vi "Auton.vi"(11 "Auton Array":dbl[][](array[numeric])) -> ()   [LabVIEW 2016]
uses:
  Robot Global Data.vi
panel:
  out "Setpoint":dbl
  out "Arg 3":dbl
  out "Arg 1":dbl=0.008
  out "Arg 2":dbl=0.00025
  out "Drive Speed":dbl
  out "Time Left":dbl
  in  "Action Variables":enum32{"Idle - 0", "Driving - 1", "Turning - 2"}(tab)
  in  "Turning Speed Bias":dbl
  in  "Min Turn Speed":dbl
  out "Turn Error":dbl
  in  "Angle Threshold":dbl=1.0
  in  "Max Turn Speed":dbl=0.3
  out "Turn Current":dbl
  out "Step Start Time":u32
  out "Step":i32
  # "Local Variables"
  # "Auton CSV (tab) Format -\n\n(Action)\\t      (Setpoint)\\t       (Timeout)\\t        (Var 1)\\t         (Var 2)\\t         (Var 3)\\t\n\n2       90       10000       0       0       0"
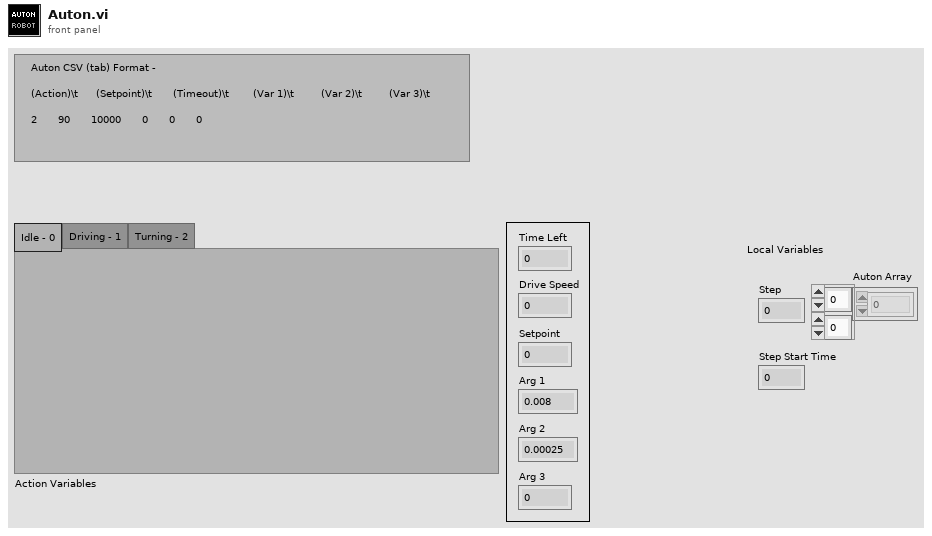
[diagram p1: front panel]
types:
  T1 = typedef "WPI_MotorControlDeviceRef.ctl" = cluster{"DeviceStatus":errorcluster, "Type":T2, "PWM":cluster{"PWM Channel":T3, "DeadBand":T4}, "CAN":cluster{"Device Number":u8, "SetOutput VI Ref":variant, "GetOutput VI Ref":variant, "Enable VI Ref":variant, "Disable VI Ref":variant, "Data":variant}, "Invert":bool}
  T2 = typedef "WPI_MotorControlType.ctl" = enum16{"PWM", "CAN"}
  T3 = typedef "FPGA_DIOPWMChannel.ctl" = enum8{"PWM 0", "PWM 1", "PWM 2", "PWM 3", "PWM 4", "PWM 5", "PWM 6", "PWM 7", "PWM 8", "PWM 9", "PWM MXP 0", "PWM MXP 1", "PWM MXP 2", "PWM MXP 3", "PWM MXP 4", "PWM MXP 5", "PWM MXP 6", "PWM MXP 7", "PWM MXP 8", "PWM MXP 9", "Invalid"}
  T4 = typedef "WPI_PWMDeadband.ctl" = cluster{"Name":string, "maxPositivePwm":i32, "minPositivePwm":i32, "centerPwm":i32, "maxNegativePwm":i32, "minNegativePwm":i32, "angularRange":u16}
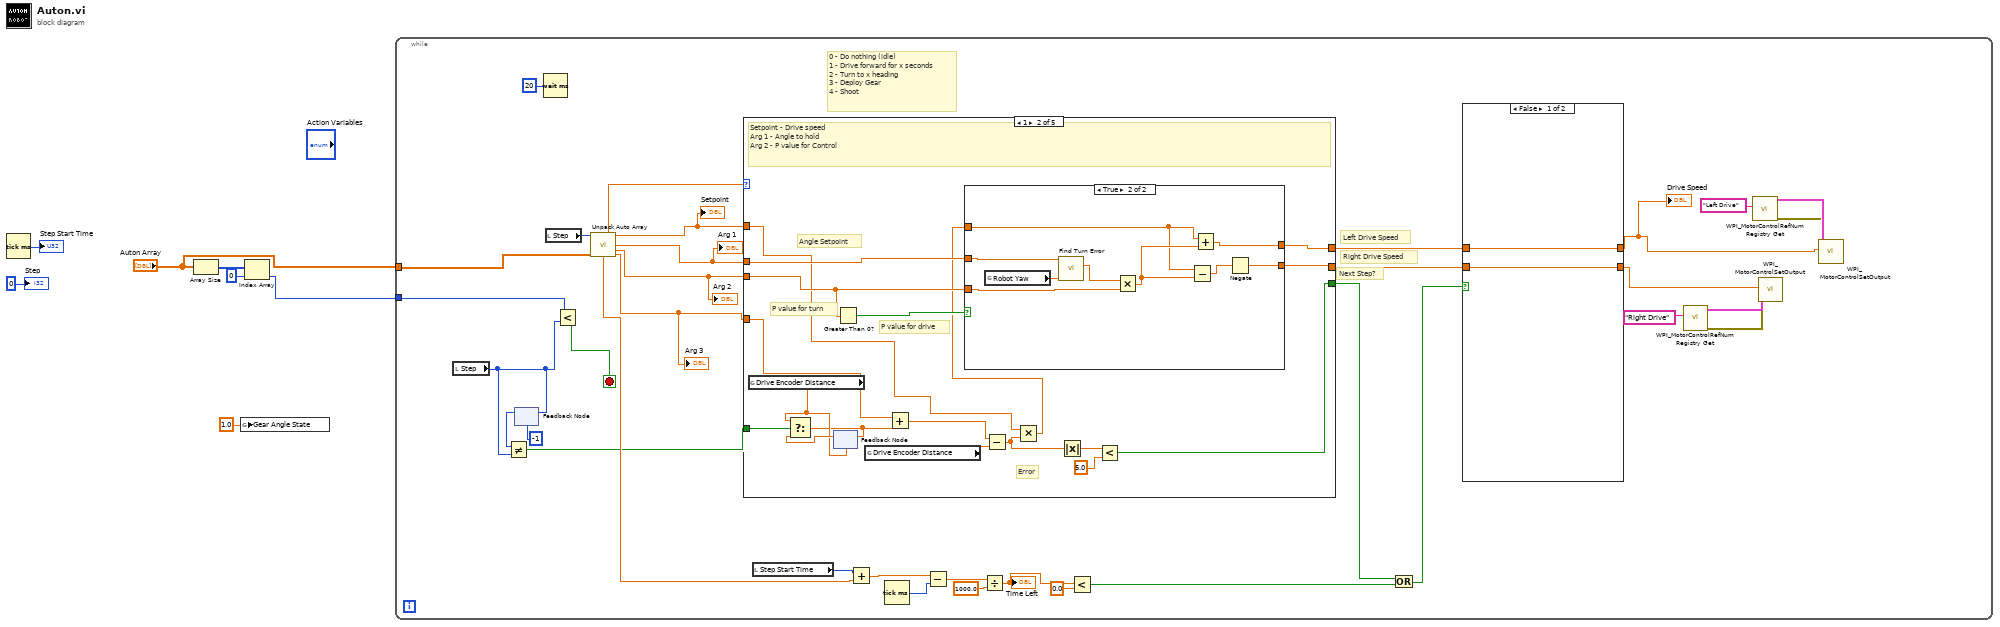
[diagram p0: block diagram]
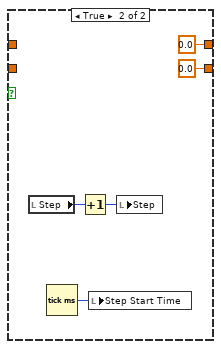
[diagram p2: hidden frame]
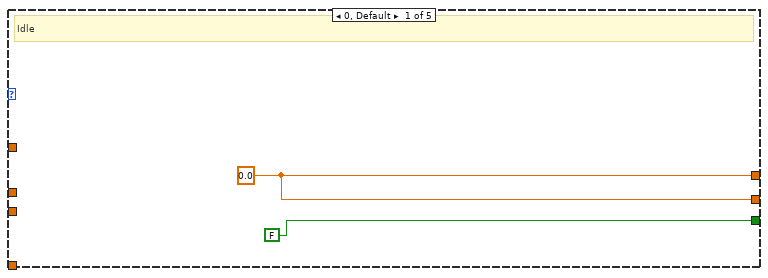
[diagram p3: hidden frame]
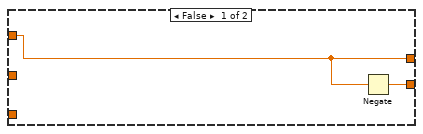
[diagram p4: hidden frame]
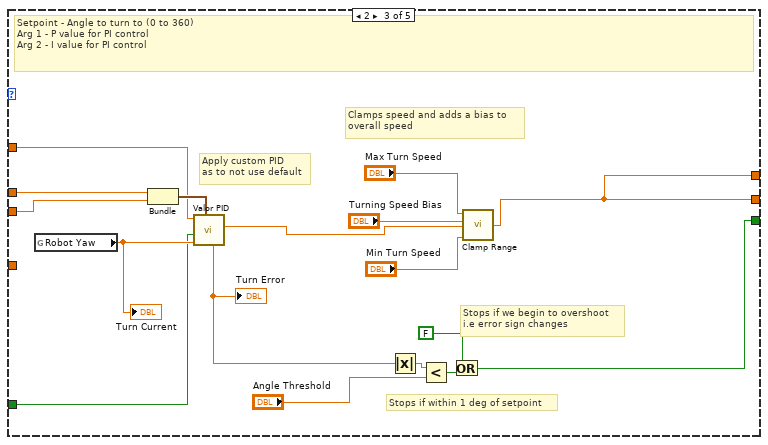
[diagram p5: hidden frame]
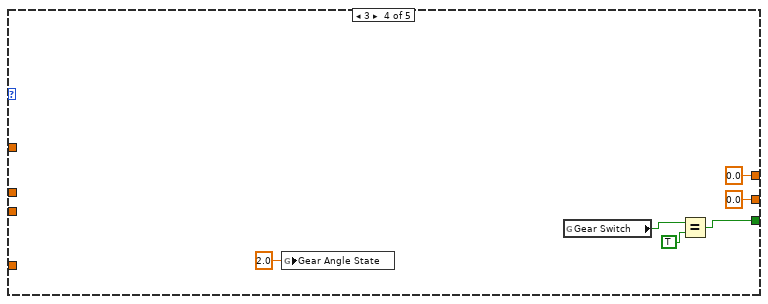
[diagram p6: hidden frame]
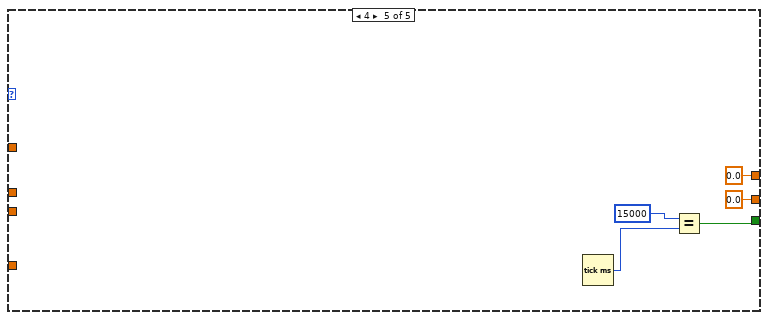
[diagram p7: hidden frame]
diagram:
  n1 = Tick Count (ms)() -> (millisecond timer value=→"Step Start Time":u32)
  n2 = Array Size(array="Auton Array") -> (size(s)=w3:i32[])
  n3 = global write "Robot Global Data.vi" "Gear Angle State"(1.0 ("Gear Angle State")) -> ()
  n4 = Index Array(array=w3, index=0) -> (element=w5:i32)
  n5 = while {
    tunnel: "Auton Array" -> [w36]
    tunnel: w5 -> [w13]
    stop <- w12 stop-if-true
    # "Next Step?"
    # "Right Drive Speed"
    # "Left Drive Speed"
    # "0 - Do nothing (idle)\n1 - Drive forward for x seconds\n2 - Turn to x heading\n3 - Deploy Gear\n4 - Shoot"
    n6 = local read "Step"() -> (w10:i32)
    n7 = feedback-in #1(w10) -> ()
    n8 = feedback #1(-1 ("Step")) -> (w11:i32)
    n9 = Not Equal?(x=w11, y=w10) -> (x != y?=w8:bool)
    n10 = Wait (ms)(milliseconds to wait=u32 20) -> ()  [unwired: 1 out]
    n11 = local read "Step"() -> (w37:i32)
    n12 = Less?(x=w13, y=w10) -> (x < y?=w12:bool)
    n13 = call "Unpack Auto Array.vi"("Step"=w37, "Auton Array"=w36) -> ("Action Type"=w35:dbl, "Setpoint"=w25:dbl, "Var 1"=w28:dbl, "Var 2"=w27:dbl, "Time Failsafe"=w29:dbl, "Var 3"=w26:dbl)  [unwired: 8 in]
    "Arg 1" <- w28
    "Arg 2" <- w27
    "Arg 3" <- w26
    "Setpoint" <- w25
    n14 = case "Auton Actions" shown="1" w35 {
      tunnel: [FALSE w52 w91 w99 w106] -> w40
      tunnel: [w50 w66 w95 0.0 ("Output") 0.0 ("Output")] -> w34
      tunnel: [w50 w65 w95 0.0 ("Output") 0.0 ("Output")] -> w38
      tunnel: w25 -> [_ w57 w83 _ _]
      tunnel: w28 -> [_ w67 w86 _ _]
      tunnel: w27 -> [_ w68 w87 _ _]
      tunnel: w26 -> [_ w61 _ _ _]
      tunnel: w8 -> [_ w64 w81 _ _]
      frame 0, Default {
        w50 = 0.0 ("Numeric")
        # "Idle"
      }
      frame 1 {
        # "Error"
        # "P value for drive"
        # "Angle Setpoint"
        # "P value for turn"
        # "Setpoint - Drive speed\nArg 1 - Angle to hold\nArg 2 - P value for Control"
        n15 = global read "Robot Global Data.vi" "Drive Encoder Distance"() -> (w62:dbl)
        n16 = feedback #2(w62) -> (w63:dbl)
        n17 = Select(t=w62, s=w64, f=w63) -> (s? t:f=w60:dbl)
        n18 = feedback-in #2(w60) -> ()
        n19 = Greater Than 0?(x=w68) -> (x > 0?=w69:bool)
        n20 = global read "Robot Global Data.vi" "Drive Encoder Distance"() -> (w58:dbl)
        n21 = Add(x=w61, y=w60) -> (x+y=w59:dbl)
        n22 = Subtract(x=w59, y=w58) -> (x-y=w55:dbl)
        n23 = Multiply(x=w57, y=w55) -> (x*y=w56:dbl)
        n24 = case shown="True" w69 {
          tunnel: w68 -> [_ w78]
          tunnel: w67 -> [_ w79]
          tunnel: [w70 w76] -> w66
          tunnel: [w71 w75] -> w65
          tunnel: w56 -> [w70 w72]
          frame False {
            n25 = Negate(x=w70) -> (-x=w71:dbl)
          }
          frame True {
            n26 = global read "Robot Global Data.vi" "Robot Yaw"() -> (w80:dbl)
            n27 = call "Find Turn Error.vi"("Target Angle"=w79, "Current Angle"=w80) -> ("Error"=w77:dbl)  [unwired: 7 in]
            n28 = Multiply(x=w77, y=w78) -> (x*y=w74:dbl)
            n29 = Subtract(x=w72, y=w74) -> (x-y=w73:dbl)
            n30 = Add(x=w72, y=w74) -> (x+y=w76:dbl)
            n31 = Negate(x=w73) -> (-x=w75:dbl)
          }
        }
        n32 = Absolute Value(x=w55) -> (abs(x)=w54:dbl)
        n33 = Less?(x=w54, y=5.0) -> (x < y?=w52:bool)
      }
      frame 2 {
        # "Apply custom PID\nas to not use default"
        # "Clamps speed and adds a bias to \noverall speed"
        # "Stops if within 1 deg of setpoint"
        # "Stops if we begin to overshoot\ni.e error sign changes"
        # "Setpoint - Angle to turn to (0 to 360)\nArg 1 - P value for PI control\nArg 2 - I value for PI control"
        n34 = global read "Robot Global Data.vi" "Robot Yaw"() -> (w90:dbl)
        "Turn Current" <- w90
        n35 = Bundle("Var 1"=w86, "Var 2"=w87) -> (w88:cluster{"Var 1":dbl, "Var 2":dbl})  [unwired: 1 in]
        n36 = call "Valor PID.vi"("PI"=w88, "Current"=w90, "First Run"=w81, "Target"=w83) -> ("Output"=w89:dbl, "Error"=w84:dbl)  [unwired: 6 in]
        "Turn Error" <- w84
        n37 = Absolute Value(x=w84) -> (abs(x)=w97:dbl)
        n38 = Less?(x=w97, y="Angle Threshold") -> (x < y?=w92:bool)
        n39 = Or(x=FALSE, y=w92) -> (x .or. y?=w91:bool)
        n40 = call "Clamp Range.vi"("Min"="Min Turn Speed", "Value"=w89, "Bias"="Turning Speed Bias", "Max"="Max Turn Speed") -> ("Output"=w95:dbl)
      }
      frame 3 {
        n41 = global write "Robot Global Data.vi" "Gear Angle State"(2.0 ("Gear Angle State")) -> ()
        n42 = global read "Robot Global Data.vi" "Gear Switch"() -> (w101:bool)
        n43 = Equal?(x=w101, y=TRUE) -> (x = y?=w99:bool)
      }
      frame 4 {
        n44 = Tick Count (ms)() -> (millisecond timer value=w105:u32)
        n45 = Equal?(x=u32 15000, y=w105) -> (x = y?=w106:bool)
      }
    }
    n46 = local read "Step Start Time"() -> (w41:u32)
    n47 = Add(x=w41, y=w29) -> (x+y=w33:dbl)
    n48 = Tick Count (ms)() -> (millisecond timer value=w32:u32)
    n49 = Subtract(x=w33, y=w32) -> (x-y=w31:dbl)
    n50 = Divide(x=w31, y=1000.0) -> (x/y=w16:dbl)
    "Time Left" <- w16
    n51 = Less?(x=w16, y=0.0) -> (x < y?=w14:bool)
    n52 = Or(x=w40, y=w14) -> (x .or. y?=w39:bool)
    n53 = case shown="False" w39 {
      tunnel: [w44 0.0 ("output")] -> w21
      tunnel: w34 -> [w44 _]
      tunnel: [w43 0.0 ("output")] -> w17
      tunnel: w38 -> [w43 _]
      frame False {
      }
      frame True {
        n54 = local read "Step"() -> (w48:i32)
        n55 = Tick Count (ms)() -> (millisecond timer value=w49:u32)
        n56 = Increment(x=w48) -> (x+1=w47:i32)
        n57 = local write "Step Start Time"(w49) -> ()
        n58 = local write "Step"(w47) -> ()
      }
    }
    "Drive Speed" <- w21
    n59 = call <vilib>:"WPI_MotorControlRefNum Registry Get.vi"("refnum name"="Right Drive") -> ("error out"=w19:errorcluster, "MotorControlDevRef"=w20:T1)  [unwired: 9 in]
    n60 = call <vilib>:"WPI_MotorControlRefNum Registry Get.vi"("refnum name"="Left Drive") -> ("error out"=w23:errorcluster, "MotorControlDevRef"=w24:T1)  [unwired: 9 in]
    n61 = call <vilib>:"WPI_MotorControlSetOutput.vi"("error in (no error)"=w19, "Output"=w17, "MotorControlDevRef"=w20) -> ()  [unwired: 6 in, 3 out]
    n62 = call <vilib>:"WPI_MotorControlSetOutput.vi"("error in (no error)"=w23, "Output"=w21, "MotorControlDevRef"=w24) -> ()  [unwired: 6 in, 3 out]
  }
  "Step" <- i8 0 ("Step")
